vi "Test Enable Plugins.vi"(8 "error in (no error)":errorcluster, 11 "Configuration Manager Test in":refnum<class "Configuration Manager Test.lvclass">) -> (0 "error out":errorcluster, 3 "Configuration Manager Test out":refnum<class "Configuration Manager Test.lvclass">)   [LabVIEW 2020, in "Configuration Manager Test.lvclass"]
uses:
  Configuration Manager Test.lvclass
  C:/Program Files (x86)/National Instruments/LabVIEW 2020/vi.lib/Astemes/LUnit/Core/LUnit Test Case/Test Case.lvclass
  <vilib>/Astemes/LUnit/Core/LUnit Test Case/Test Case.lvclass/Test Case.ctl
  b78b68b9-28ec-4fcb-9b61-f705c7f0904e.vi
  <vilib>/Astemes/LUnit/Core/LUnit Test Case/Private/Append Pass Result.vi
  <vilib>/Astemes/LUnit/Core/LUnit Test Case/Private/Append Fail Result.vi
  b78b68b9-28ec-4fcb-9b61-f705c7f0904e.vi/9c5d11cd-9439-4240-a1ee-d9baace9c924.vi
  <vilib>/Astemes/LUnit/Core/LUnit Test Case/Private/Run In UI.vi
  <vilib>/Utility/error.llb/Clear Errors.vi
  source/User Interface/Configuration Manager/Configuration Manager.lvclass
panel:
  out "Array":string[](array[string])=["tets.lvclass", "disabled.lvclass "]
  out "Plugins":string[](array[string])
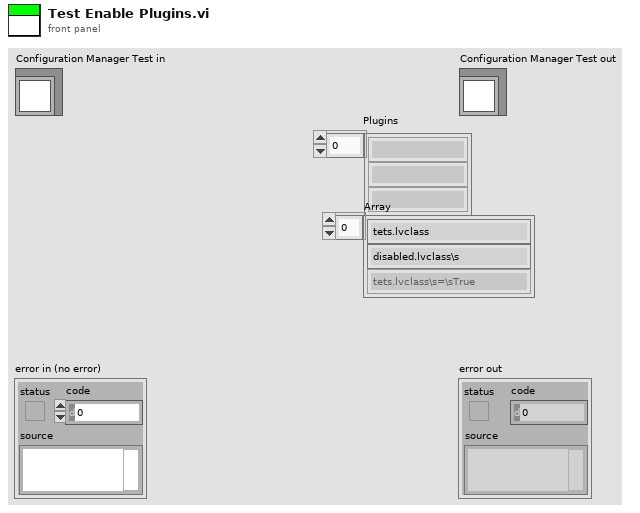
[diagram p1: front panel]
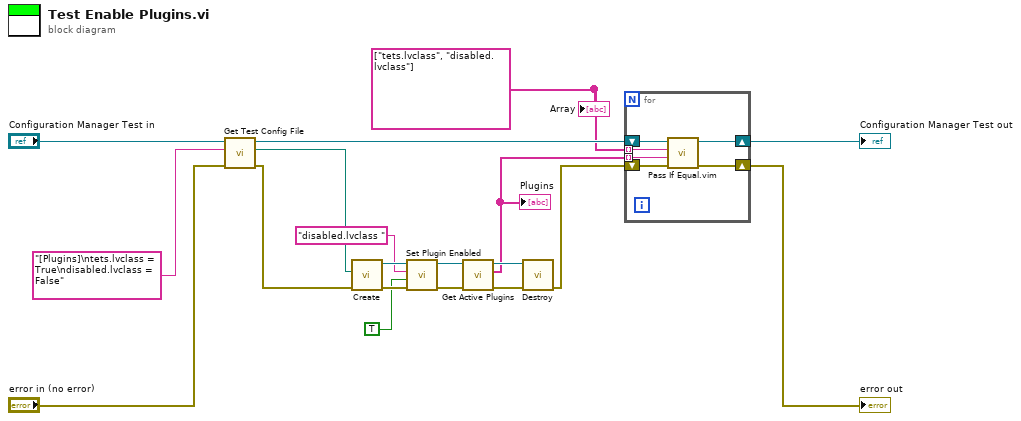
[diagram p0: block diagram]
diagram:
  w7 = string[] ["tets.lvclass", "disabled.lvclass"]
  n1 = call "Get Test Config File.vi"("error in (no error)"="error in (no error)", "File Content"="[Plugins]\ntets.lvclass = True\ndisabled.lvclass = False", "Configuration Manager Test in"="Configuration Manager Test in") -> ("error out"=w13:errorcluster, "File Path"=w8:path, "Configuration Manager Test out"=w10:refnum<class "Configuration Manager Test.lvclass">)  [unwired: 6 in]
  n2 = call "Create.vi"("error in (no error)"=w13, "configuration file path"=w8) -> ("error out"=w16:errorcluster, "Configuration Manager out"=w5:refnum<class "Configuration Manager.lvclass">)  [unwired: 8 in]
  n3 = call "Set Plugin Enabled.vi"("error in (no error)"=w16, "Enabled?"=TRUE, "Plugin"="disabled.lvclass ", "Configuration Manager in"=w5) -> ("error out"=w6:errorcluster, "Configuration Manager out"=w4:refnum<class "Configuration Manager.lvclass">)  [unwired: 6 in]
  n4 = call "Get Active Plugins.vi"("error in (no error)"=w6, "Configuration Manager In"=w4) -> ("error out"=w14:errorcluster, "Plugins"=w1:string[], "Configuration Manager Out"=w15:refnum<class "Configuration Manager.lvclass">)  [unwired: 7 in]
  "Plugins" <- w1
  n5 = call "Destroy.vi"("error in (no error)"=w14, "Configuration Manager In"=w15) -> ("error out"=w12:errorcluster)  [unwired: 9 in]
  n6 = for {
    tunnel: w7 -> [w21] mode=indexing
    tunnel: w1 -> [w20] mode=indexing
    shift-right: [w24] -> w11
    shift-left: w12 -> [w25]
    shift-right: [w22] -> w9
    shift-left: w10 -> [w23]
    n7 = call "Pass If Equal.vim"("error in (no error)"=w25, "Actual"=w20, "Expected"=w21, "LUnit Test Case In"=w23) -> ("error out"=w24:errorcluster, "LUnit Test Case Out"=w22:refnum<class "Configuration Manager Test.lvclass">)  [unwired: 6 in]
  }
  "error out" <- w11
  "Configuration Manager Test out" <- w9
  "Array" <- w7
